vi "calcsignalcontinous.vi"() -> ()   [LabVIEW 2019]
uses:
  ExperimentSeries_class/ExperimentSeries.lvclass
  <vilib>/gmath/NI_Gmath.lvlib
panel:
  out "Array":dbl[](array[numeric])=[9.991620709231703e-08, 9.608358822859203e-08, 9.442919915695634e-08, 9.847044704615725e-08, 9.317262744074929e-08]
  out "XY Graph":cluster{dbl[], sgl[]}[](graph)=[{array[203 elements], [0.0, 0.0121169835, 0.012025846, 0.013386696, 0.013375319, 0.013415199, 0.014776048, 0.015504916, 0.018426016, 0.022690842, 0.02587386, 0.032319542, 0.03677802, 0.04455042, 0.051611073, 0.059628382, 0.06832319, 0.07868075, 0.089510895, 0.10068272, 0.11326654, 0.12563981, 0.14052412, 0.15370591, 0.16707559, 0.18078697, 0.1960642, 0.21136984, 0.22496732, 0.24160542, 0.2562563, 0.2698025, 0.28704423, 0.3018944, 0.31668758, 0.3310993, 0.34738433, 0.36231992, 0.37776795, 0.393347, 0.40835658, 0.42209643, 0.43828472, 0.4511931, 0.46653298, 0.4809732, 0.4951799, 0.50926137, 0.52341115, 0.537914, 0.5514317, 0.56353164, 0.576628, 0.58912086, 0.60132325, 0.61523384, 0.6256028, 0.63757175, 0.64855564, 0.6607125, 0.6710359, 0.68158126, 0.69270754, 0.702285, 0.71166885, 0.72137153, 0.7306415, 0.7391598, 0.74926114, 0.7569083, 0.76519316, 0.7719919, 0.7796903, 0.7866086, 0.7937831, 0.8002687, 0.806555, 0.8132398, 0.8201012, 0.82628495, 0.8333912, 0.8390568, 0.8442953, 0.8503595, 0.8550572, 0.8606089, 0.8666104, 0.8714048, 0.87658644, 0.88064635, 0.8861525, 0.89004725, 0.89486444, 0.8988731, 0.9024433, 0.90729463, 0.91087055, 0.91478807, 0.91881377, 0.9232039, 0.9266602, 0.9301962, 0.93421626, 0.9370063, 0.9407303, 0.94526273, 0.9479048, 0.95276755, 0.95632637, 0.95901966, 0.9615991, 0.96448034, 0.96679777, 0.9699181, 0.97130746, 0.97489476, 0.9762157, 0.9789262, 0.98026997, 0.982912, 0.9846316, 0.98604375, 0.98735344, 0.98901606, 0.99073, 0.990878, 0.9932638, 0.9958091, 0.9966632, 0.9974205, 0.99954444, 0.999254, 1.0012527, 1.0013893, 1.0035473, 1.0040085, 1.0036783, 1.0048968, 1.0058478, 1.0066905, 1.0076128, 1.0084897, 1.00964, 1.0101867, 1.0105283, 1.0120087, 1.0121682, 1.0125896, 1.0130223, 1.0141041, 1.0135405, 1.0142181, 1.0145938, 1.0143946, 1.0148785, 1.0149584, 1.0150095, 1.0144913, 1.0145426, 1.0151006, 1.0141497, 1.0134096, 1.0130166, 1.0123447, 1.0122821, 1.0120145, 1.0114167, 1.0106194, 1.0102607, 1.0100273, 1.0101354, 1.0098051, 1.0098336, 1.0090307, 1.0089453, 1.00886, 1.0082963, 1.0079318, 1.007129, 1.0076357, 1.006867, 1.0074819, 1.0067588, 1.0066677, 1.0064172, 1.0059502, 1.0050336, 1.005119, 1.0046293, 1.0044129, 1.0036157, 1.0037183, 1.0042078, 1.0038377, 1.0030919, 1.0023516, 1.0021807, 1.0013893, 1.0000341, 1.0003587, 1.000239, 1.0020328, 1.0]}, {array[206 elements], [0.0, 0.013095012, 0.009945136, 0.007707864, 0.008644557, 0.0078271935, 0.00842384, 0.00935451, 0.011466431, 0.013494784, 0.016453808, 0.02358309, 0.029948715, 0.037059933, 0.044582963, 0.054140247, 0.06453284, 0.074137926, 0.084918246, 0.09915285, 0.108883165, 0.12211545, 0.13460805, 0.14785224, 0.16131729, 0.17449586, 0.18805037, 0.2017778, 0.2144374, 0.22796205, 0.24115254, 0.25469515, 0.26897743, 0.28243643, 0.29761952, 0.31075042, 0.32516408, 0.33873641, 0.3513841, 0.36468202, 0.3790895, 0.3934792, 0.4062343, 0.42070755, 0.43550888, 0.4477031, 0.46219423, 0.4754564, 0.48988184, 0.5039553, 0.5169311, 0.53081965, 0.5443443, 0.5583522, 0.5718112, 0.5844827, 0.5980551, 0.6100763, 0.6219544, 0.6346617, 0.6460506, 0.6576005, 0.66909075, 0.6800501, 0.69037104, 0.70170027, 0.7118959, 0.72204983, 0.7321322, 0.7410153, 0.7503221, 0.76020163, 0.7683271, 0.77725804, 0.7855506, 0.79396844, 0.8013005, 0.8097005, 0.8171996, 0.8252535, 0.831291, 0.8380086, 0.8446008, 0.8515034, 0.8570695, 0.86343515, 0.8674621, 0.8741916, 0.8789762, 0.88484067, 0.8897983, 0.89425486, 0.897894, 0.90239227, 0.90657437, 0.9113888, 0.9146641, 0.9192936, 0.9221274, 0.92619014, 0.9297816, 0.93324775, 0.9365052, 0.93976253, 0.94276935, 0.94702893, 0.9495466, 0.9533707, 0.95685476, 0.9595871, 0.96235526, 0.964688, 0.9683808, 0.9693592, 0.9722169, 0.9743765, 0.9773595, 0.97899413, 0.981458, 0.9836236, 0.9847333, 0.9867259, 0.98960143, 0.9906574, 0.9919818, 0.99466056, 0.9960685, 0.9973213, 0.99933773, 1.0002625, 1.0003937, 1.0031141, 1.0044087, 1.0057272, 1.0072724, 1.0066878, 1.0081732, 1.0092947, 1.011007, 1.0114664, 1.0116991, 1.0118362, 1.0133098, 1.0137274, 1.0149325, 1.016072, 1.0156723, 1.0165136, 1.0161616, 1.0168834, 1.0164717, 1.016263, 1.0154994, 1.0154098, 1.016245, 1.0145985, 1.0145924, 1.0143241, 1.0137632, 1.0127132, 1.0137036, 1.013459, 1.0123553, 1.0118542, 1.0123373, 1.0117646, 1.0110248, 1.0111502, 1.0108519, 1.010482, 1.0101061, 1.0100226, 1.0103985, 1.0090203, 1.0091754, 1.0092888, 1.0087638, 1.008728, 1.0084476, 1.0087698, 1.0084596, 1.0095632, 1.0088772, 1.0088772, 1.0088295, 1.0080479, 1.0077795, 1.0068488, 1.0074753, 1.0071292, 1.0064491, 1.0068429, 1.0067116, 1.0077795, 1.006109, 1.0059301, 1.0060135, 1.0046772, 1.0037704, 1.0046712, 1.0029709, 1.0029113, 1.0014378, 1.0015988, 1.0016824, 1.0]}, {array[210 elements], [0.0, 0.007065828, 0.005442325, 0.0054787756, 0.004864623, 0.0042321817, 0.0032349816, 0.002091853, 0.0030281763, 0.0050531398, 0.008026702, 0.0110731665, 0.016351275, 0.019647008, 0.026354214, 0.031072909, 0.03716584, 0.0470836, 0.054137405, 0.06389095, 0.072525665, 0.08295424, 0.095523275, 0.10713769, 0.12001674, 0.13320605, 0.14600006, 0.15848391, 0.17093745, 0.18463132, 0.19852598, 0.21247539, 0.22754362, 0.24159636, 0.25617206, 0.27060786, 0.28604096, 0.30135232, 0.3165179, 0.33310628, 0.348363, 0.36489668, 0.38134527, 0.39616424, 0.41173106, 0.4275533, 0.44350326, 0.45896065, 0.47438765, 0.48806942, 0.5031255, 0.5178168, 0.5310668, 0.5446331, 0.5584304, 0.5723737, 0.5851494, 0.5977185, 0.610926, 0.6221754, 0.6341547, 0.6471067, 0.65757185, 0.6690767, 0.68011945, 0.69166684, 0.702138, 0.7115511, 0.721554, 0.7311738, 0.74081796, 0.749854, 0.75840366, 0.766558, 0.77403736, 0.7815046, 0.78883195, 0.79684037, 0.8040279, 0.8116715, 0.819315, 0.8251283, 0.8315678, 0.8380439, 0.8440882, 0.8514764, 0.85626805, 0.8633218, 0.86940265, 0.8744922, 0.8804575, 0.8852249, 0.8911415, 0.8962919, 0.89983094, 0.9062583, 0.9103021, 0.91511196, 0.91969085, 0.92488384, 0.9292924, 0.93225986, 0.9353732, 0.937988, 0.94204384, 0.94629437, 0.95065427, 0.9526062, 0.9555737, 0.95924646, 0.96222603, 0.9653698, 0.9675893, 0.97107357, 0.97311676, 0.97565246, 0.9783584, 0.9808941, 0.9830163, 0.98448783, 0.98680466, 0.98964435, 0.98951054, 0.9902889, 0.9924902, 0.99390095, 0.99463063, 0.9965035, 0.99730015, 0.99812096, 0.9990027, 1.00121, 1.0019579, 1.0034478, 1.0046396, 1.0052903, 1.0054909, 1.0064821, 1.0075524, 1.0081605, 1.0083793, 1.009261, 1.010167, 1.0097597, 1.0106171, 1.0105197, 1.0108786, 1.0114563, 1.0114563, 1.0116751, 1.0124778, 1.0117116, 1.0122163, 1.0115474, 1.0117359, 1.0119002, 1.0118697, 1.0114866, 1.0117055, 1.0114988, 1.0110184, 1.0106778, 1.0108056, 1.0099603, 1.0108237, 1.0099664, 1.009936, 1.0103313, 1.0104164, 1.0102766, 1.0099785, 1.0102948, 1.0093704, 1.0088718, 1.0093644, 1.0090239, 1.0085678, 1.0080144, 1.006932, 1.0068226, 1.0078564, 1.0070416, 1.0058193, 1.0053511, 1.0042322, 1.0055456, 1.0047247, 1.0056368, 1.0046275, 1.0037154, 1.0041288, 1.0033991, 1.0030829, 1.002189, 1.0012283, 1.0013682, 1.0005716, 1.0001459, 1.0001277, 1.0005047, 1.000906, 1.0012466, 1.0006932, 1.0008999, 1.0003223, 1.0010884, 1.0020249, 1.0010276, 1.0016844, 1.0]}, {array[205 elements], [0.0, 0.010129304, 0.012169545, 0.011816631, 0.015196738, 0.017656, 0.02093138, 0.023815228, 0.028750334, 0.033123072, 0.0382732, 0.04141625, 0.045915753, 0.053773213, 0.06118973, 0.06957105, 0.07907733, 0.08785575, 0.09808444, 0.10974671, 0.12112774, 0.13315393, 0.14552748, 0.15823747, 0.17151539, 0.18441279, 0.19857295, 0.21374765, 0.2277148, 0.24101476, 0.256173, 0.26996922, 0.28457054, 0.30083704, 0.31490892, 0.33066815, 0.34488904, 0.35923117, 0.3731101, 0.3879815, 0.40296322, 0.41513288, 0.42929304, 0.44358552, 0.45790002, 0.47278252, 0.4868048, 0.50061756, 0.51429796, 0.52865666, 0.54119015, 0.5546776, 0.5666266, 0.57986593, 0.5918425, 0.6036095, 0.6156192, 0.6276674, 0.63955027, 0.6501097, 0.66070783, 0.6717966, 0.68332106, 0.69312507, 0.70354116, 0.71304744, 0.72300035, 0.73193866, 0.74170965, 0.75154674, 0.7605071, 0.76894915, 0.7772589, 0.7853866, 0.7936357, 0.7992766, 0.8072665, 0.813922, 0.82100207, 0.82743144, 0.8338609, 0.83992636, 0.84513164, 0.8508718, 0.85644656, 0.8624128, 0.86609066, 0.87152755, 0.8757844, 0.88063127, 0.8844691, 0.88891345, 0.8941077, 0.8979841, 0.902456, 0.9058747, 0.9102198, 0.91389775, 0.91843027, 0.9214189, 0.92441857, 0.92832255, 0.93139386, 0.9342171, 0.9366929, 0.9391301, 0.9433153, 0.9456643, 0.9474178, 0.95010316, 0.95237494, 0.95469093, 0.9567034, 0.96008366, 0.9614677, 0.962405, 0.9655095, 0.9683106, 0.96936935, 0.9711834, 0.9723635, 0.9746794, 0.9763998, 0.979245, 0.98064566, 0.9821785, 0.9838052, 0.984693, 0.9869813, 0.98791873, 0.9894736, 0.9909018, 0.99207634, 0.99340516, 0.99446934, 0.9958314, 0.9959969, 0.99655926, 0.99739194, 0.9977613, 0.998434, 0.9996803, 0.99966913, 1.0004191, 1.0017977, 1.0017259, 1.0024868, 1.0033802, 1.003733, 1.0035952, 1.003904, 1.0034353, 1.0044057, 1.0056299, 1.0053266, 1.00531, 1.0061978, 1.0062971, 1.0060159, 1.0069534, 1.0065287, 1.0069036, 1.0065894, 1.0072014, 1.007047, 1.0071297, 1.0069534, 1.0073669, 1.007047, 1.0075874, 1.0077362, 1.0081388, 1.0069534, 1.00858, 1.0087839, 1.0087067, 1.0073006, 1.008762, 1.0075874, 1.0080671, 1.0083594, 1.0076866, 1.0078025, 1.0074606, 1.0077803, 1.0076536, 1.007455, 1.0066501, 1.0062034, 1.0061538, 1.007047, 1.0064294, 1.0062311, 1.0057071, 1.0054259, 1.0054755, 1.0053487, 1.0046539, 1.0041522, 1.0027626, 1.0035787, 1.0032754, 1.0018859, 1.0018748, 1.0]}, {array[209 elements], [0.0, 0.008427129, 0.00952319, 0.009181468, 0.010118382, 0.011338264, 0.012316573, 0.0131473895, 0.01614702, 0.019588523, 0.024250029, 0.02864617, 0.033908695, 0.039259594, 0.04668486, 0.05362104, 0.061723925, 0.06842435, 0.07814796, 0.087959945, 0.097571515, 0.11055393, 0.12145603, 0.13384324, 0.14762127, 0.16086894, 0.17325616, 0.18685137, 0.19920921, 0.21327592, 0.22729552, 0.24081425, 0.25439185, 0.26848212, 0.2820715, 0.29479462, 0.3086434, 0.32273367, 0.33718348, 0.35061967, 0.36488083, 0.37923634, 0.39437568, 0.4086781, 0.42145428, 0.4350614, 0.4489101, 0.4627588, 0.47694927, 0.49004367, 0.504022, 0.5165153, 0.5301755, 0.5424331, 0.5554096, 0.56681263, 0.5795358, 0.5915694, 0.60262483, 0.61440504, 0.6252011, 0.636062, 0.647141, 0.65834373, 0.66843855, 0.67858636, 0.68932945, 0.69833994, 0.70862925, 0.71781653, 0.7267622, 0.7348475, 0.74316263, 0.7512597, 0.7602112, 0.76750684, 0.7755273, 0.78279936, 0.7908198, 0.7975025, 0.8039849, 0.81126285, 0.8187353, 0.8234615, 0.8305391, 0.8375577, 0.8433506, 0.8483302, 0.8541761, 0.8599455, 0.86542016, 0.8698988, 0.875291, 0.8801233, 0.8835177, 0.8889217, 0.8926343, 0.8966828, 0.9001126, 0.9043615, 0.9087872, 0.912052, 0.9161299, 0.9195479, 0.9225828, 0.92705566, 0.93083316, 0.93393874, 0.9363608, 0.94027376, 0.94383323, 0.9456188, 0.9475576, 0.9504865, 0.9539457, 0.9554661, 0.9580178, 0.960375, 0.96305054, 0.9655256, 0.9673289, 0.9699277, 0.9723026, 0.974318, 0.97704065, 0.9779482, 0.97999305, 0.98229724, 0.9833934, 0.9854206, 0.9864872, 0.98711777, 0.9892864, 0.99112505, 0.9907774, 0.99285173, 0.99289304, 0.9943545, 0.993777, 0.9945666, 0.99647003, 0.99777836, 0.99911606, 1.0003595, 1.0006717, 1.0009784, 1.0025694, 1.0030938, 1.0044198, 1.0041252, 1.0051211, 1.0053568, 1.0063232, 1.0061111, 1.0065767, 1.0073723, 1.0079969, 1.0073899, 1.0077258, 1.0090812, 1.0086156, 1.0095762, 1.0082384, 1.0086864, 1.009806, 1.0097, 1.0090812, 1.0101007, 1.0097119, 1.0100477, 1.0095645, 1.0101243, 1.0095409, 1.0099652, 1.0103658, 1.0106429, 1.0109847, 1.010743, 1.0106547, 1.0100241, 1.0094584, 1.009535, 1.0097237, 1.0088986, 1.0085567, 1.0083799, 1.0087631, 1.0081913, 1.0075549, 1.0066946, 1.0062938, 1.0070245, 1.0052803, 1.0051976, 1.0039778, 1.0045081, 1.0045141, 1.0044376, 1.0034592, 1.0039307, 1.0037009, 1.002263, 1.0027344, 1.0026107, 1.001373, 1.002157, 1.0011315, 1.0006837, 1.0]}]
  in  "dt(s)":dbl=0.1
  in  "Frequency":dbl=1770000.0
  in  "directory path":path=path "D:/pulsed/continous/1,77mhz0,3V"
  in  "ThresholdRange":cluster{"Lower value":sgl, "Upper value":sgl}={"Lower value"=800.0, "Upper value"=500000.0} {"Upper value" format="%.2f"; "Lower value" format="%.2f"}
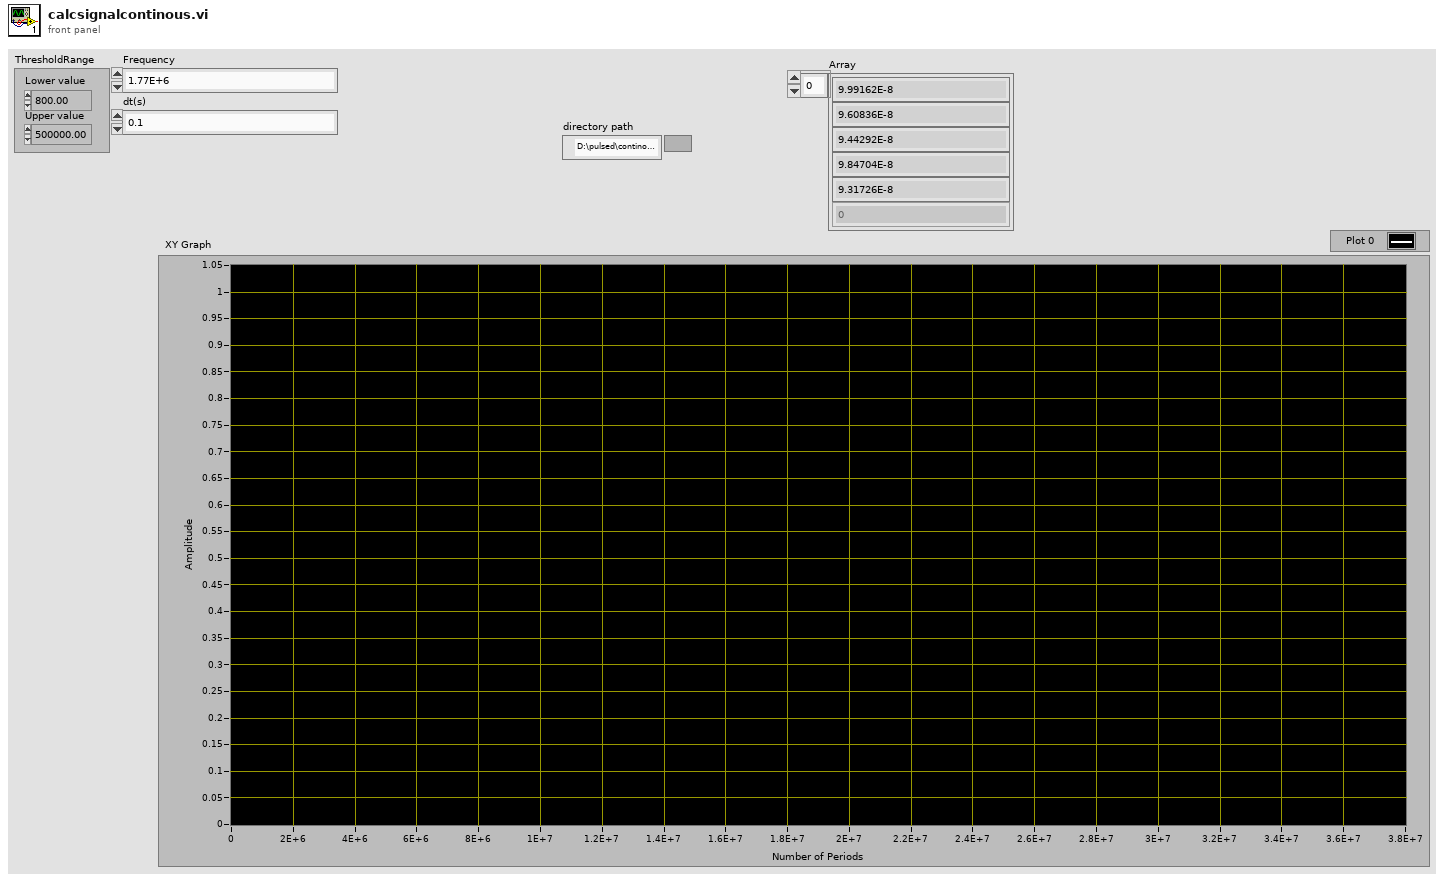
[diagram p1: front panel]
types:
  T1 = typedef "Image Type" = u32
  T2 = typedef "IMAQ Image.ctl" = refnum<image>
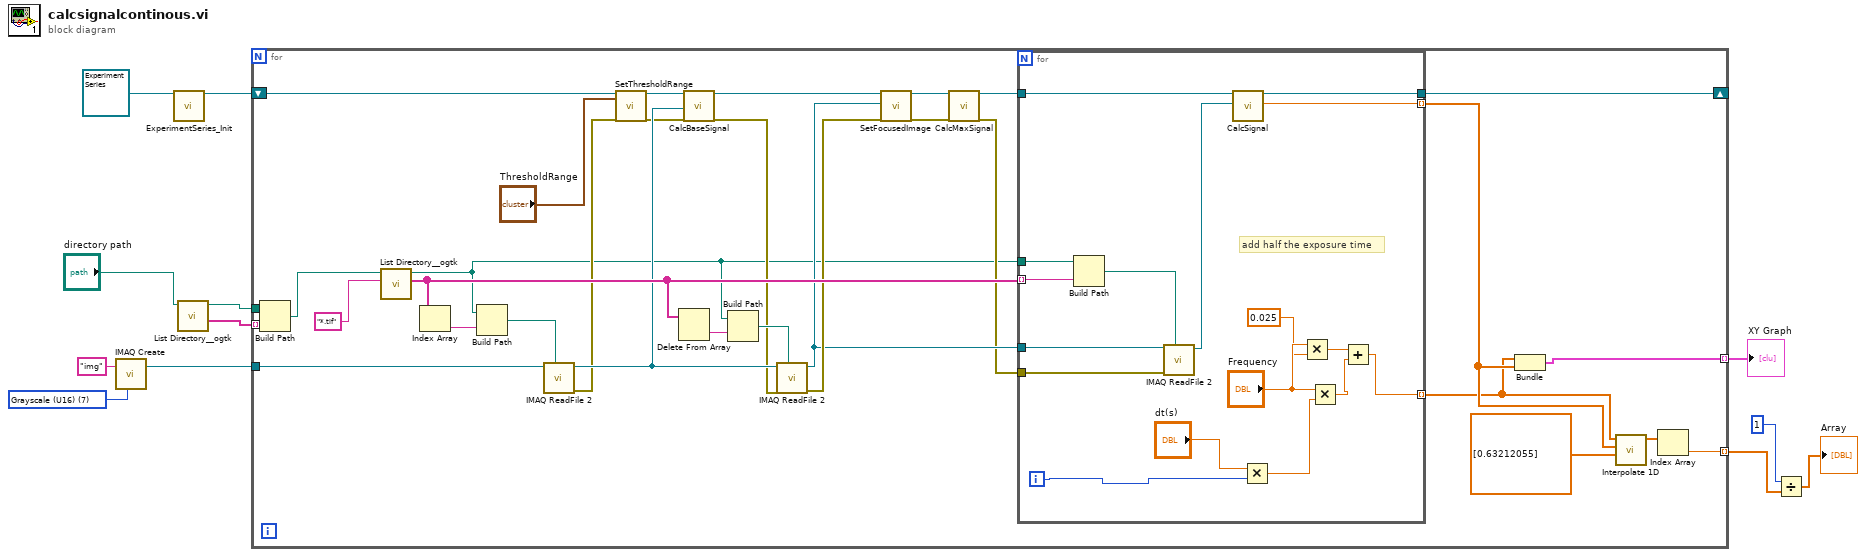
[diagram p0: block diagram]
diagram:
  w2 = T1 7 items=["Grayscale (U8)", "Grayscale (I16)", "Grayscale (SGL)", "Complex (CSG)", "RGB (U32)", "HSL (U32)", "RGB (U64)", "Grayscale (U16)"] ("Image Type")
  n1 = call "IMAQ Create"("Image Name"="img", "Image Type"=w2) -> ("New Image"=w1:T2)  [unwired: 3 in, 1 out]
  n2 = call "ExperimentSeries_Init.vi"("object in"=refnum<class "ExperimentSeries.lvclass"> refnum) -> ("object out"=w11:refnum<class "ExperimentSeries.lvclass">)  [unwired: 17 in, 1 out]
  n3 = call <userlib>:"List Directory__ogtk.vi"("directory path"="directory path") -> ("directory names"=w9:string[], "dup directory path"=w10:path)  [unwired: 3 in, 2 out]
  n4 = for {
    tunnel: [w21] -> w6 mode=indexing
    tunnel: w10 -> [w19]
    tunnel: w9 -> [w18] mode=indexing
    tunnel: [w16] -> w7 mode=indexing
    tunnel: w1 -> [w15]
    shift-right: [w14] -> _
    shift-left: w11 -> [w40]
    n5 = Build Path(base path=w19, name or relative path=w18) -> (appended path=w17:path)
    n6 = call <userlib>:"List Directory__ogtk.vi"("pattern"="*.tif", "directory path"=w17) -> ("file names"=w37:string[], "dup directory path"=w24:path)  [unwired: 2 in, 2 out]
    n7 = Index Array(array=w37) -> (element=w39:string)  [unwired: 1 in]
    n8 = Build Path(base path=w24, name or relative path=w39) -> (appended path=w35:path)
    n9 = call "IMAQ ReadFile 2"("File Path"=w35, "Image"=w15) -> ("error out"=w33:errorcluster, "Image Out"=w34:T2)  [unwired: 5 in, 3 out]
    n10 = call-dynamic "SetThresholdRange.vi"("object in"=w40, "ThresholdRange"="ThresholdRange", "error in (no error)"=w33) -> ("object out"=w44:refnum<class "ExperimentSeries.lvclass">, "error out"=w32:errorcluster)  [unwired: 15 in]
    n11 = Delete From Array(array=w37) -> (deleted portion=w36:string)  [unwired: 2 in, 1 out]
    n12 = call-dynamic "CalcBaseSignal.vi"("object in"=w44, "First Frame"=w34, "error in (no error)"=w32) -> ("object out"=w42:refnum<class "ExperimentSeries.lvclass">, "error out"=w31:errorcluster)  [unwired: 15 in]
    n13 = Build Path(base path=w24, name or relative path=w36) -> (appended path=w38:path)
    n14 = call "IMAQ ReadFile 2"("File Path"=w38, "error in (no error)"=w31, "Image"=w34) -> ("error out"=w27:errorcluster, "Image Out"=w26:T2)  [unwired: 4 in, 3 out]
    n15 = call-dynamic "SetFocusedImage.vi"("object in"=w42, "Image"=w26, "error in (no error)"=w27) -> ("object out"=w30:refnum<class "ExperimentSeries.lvclass">, "error out"=w28:errorcluster)  [unwired: 15 in]
    n16 = call-dynamic "CalcMaxSignal.vi"("object in"=w30, "error in (no error)"=w28) -> ("object out"=w29:refnum<class "ExperimentSeries.lvclass">, "error out"=w25:errorcluster)  [unwired: 16 in]
    n17 = for {
      tunnel: w24 -> [w61]
      tunnel: w37 -> [w60] mode=indexing
      tunnel: w26 -> [w59]
      tunnel: w29 -> [w58]
      tunnel: w25 -> [w57]
      tunnel: [w47] -> w13 mode=indexing
      tunnel: [w52] -> w20 mode=indexing
      tunnel: [w51] -> w14
      i -> [w45]
      # "add half the exposure time"
      n18 = Build Path(base path=w61, name or relative path=w60) -> (appended path=w55:path)
      n19 = call "IMAQ ReadFile 2"("File Path"=w55, "error in (no error)"=w57, "Image"=w59) -> ("Image Out"=w56:T2)  [unwired: 4 in, 4 out]
      n20 = call-dynamic "CalcSignal.vi"("object in"=w58, "Current Frame"=w56) -> ("object out"=w51:refnum<class "ExperimentSeries.lvclass">, "Signal"=w52:sgl)  [unwired: 15 in, 1 out]
      n21 = Multiply(x="dt(s)", y=w45) -> (x*y=w53:dbl)
      n22 = Multiply(x="Frequency", y=0.025) -> (x*y=w49:dbl)
      n23 = Multiply(x="Frequency", y=w53) -> (x*y=w48:dbl)
      n24 = Add(x=w49, y=w48) -> (x+y=w47:dbl)
    }
    n25 = Bundle(w13, w20) -> (w16:cluster{dbl[], sgl[]})  [unwired: 1 in]
    n26 = call <vilib>:"Interpolate 1D.vi"("xi"=dbl[] [0.63212055], "X"=w20, "Y"=w13) -> ("yi"=w22:dbl[])  [unwired: 6 in, 2 out]
    n27 = Index Array(array=w22) -> (element=w21:dbl)  [unwired: 1 in]
  }
  "XY Graph" <- w7
  n28 = Divide(x=1, y=w6) -> (x/y=→"Array":dbl[])
